vi "数据查询.vi"() -> ()   [LabVIEW 2016, in "数据查询.lvlib"]
uses:
  <vilib>/Utility/miscctls.llb/LVPointTypeDef.ctl
panel:
  in  "标识说明":bool
  in  "数据查询菜单":enum32{"数据查询", "仪器数据", "仪器日志", "报警信息", "校准日志"}(xcontrol)
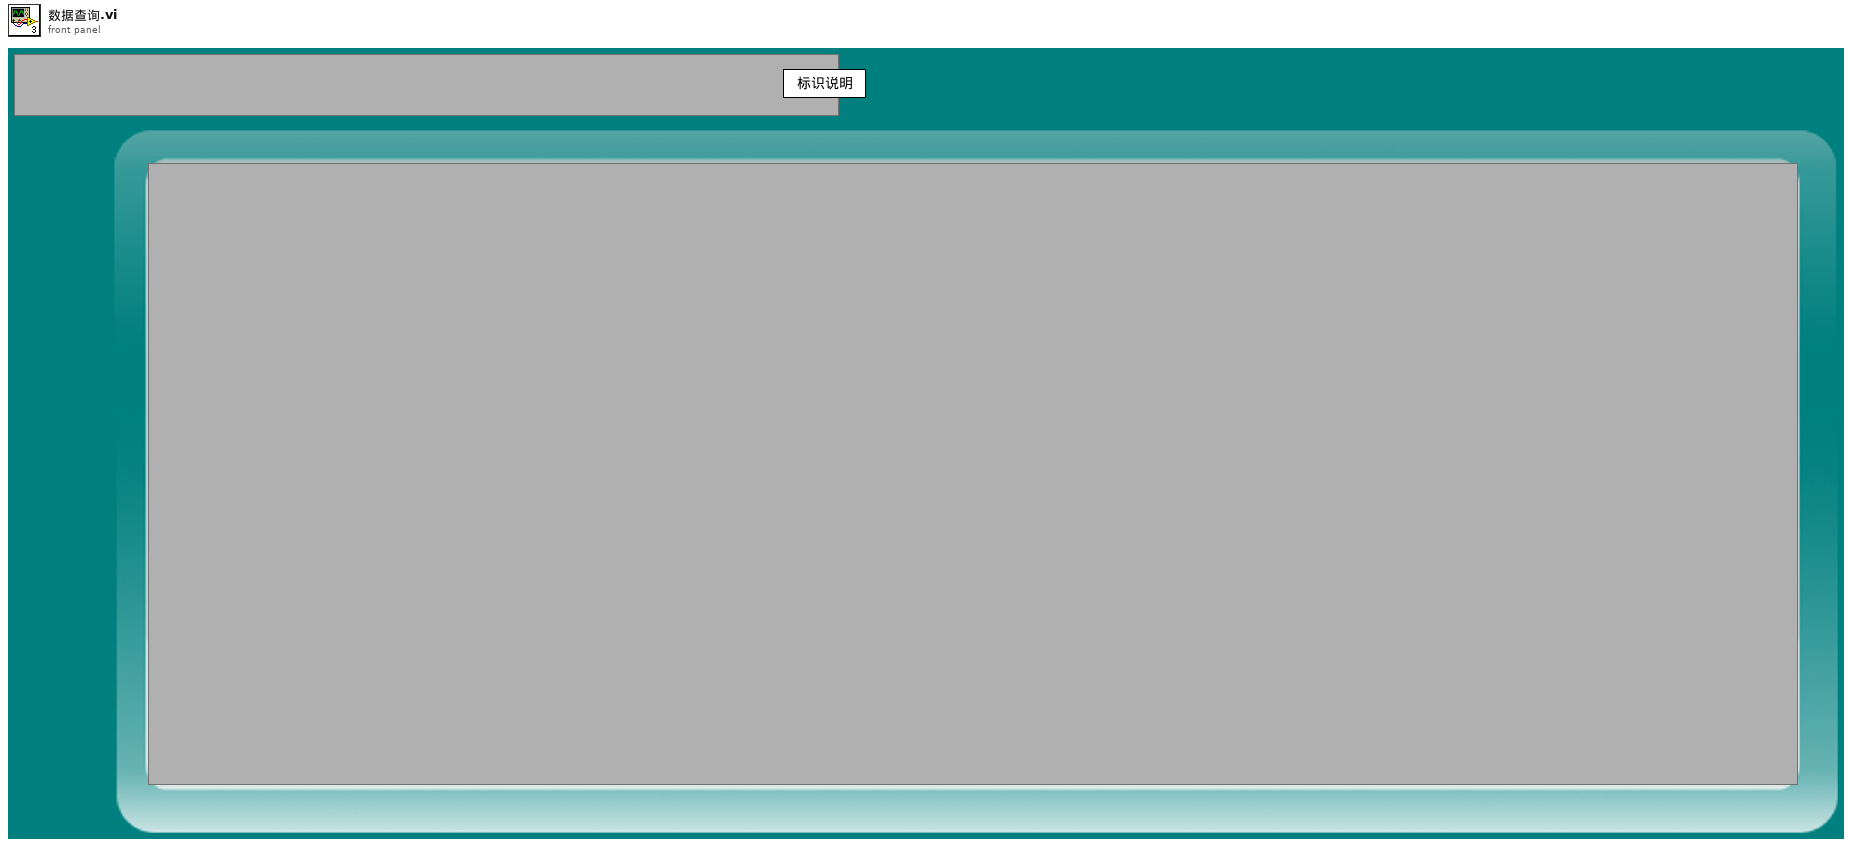
[diagram p1: front panel]
types:
  T1 = typedef "LVPointTypeDef.ctl" = cluster{"Horizontal":i16, "Vertical":i16}
  T2 = enum32{"Bad", "Idle", "Run top level", "Running"}
  T3 = typedef "LVDateTimeRec.ctl" = cluster{"秒数的小数部分":dbl, "秒":i32, "分":i32, "时":i32, "日":i32, "月":i32, "年":i32, "天数（周）":i32, "天数（年）":i32, "DST":i32}
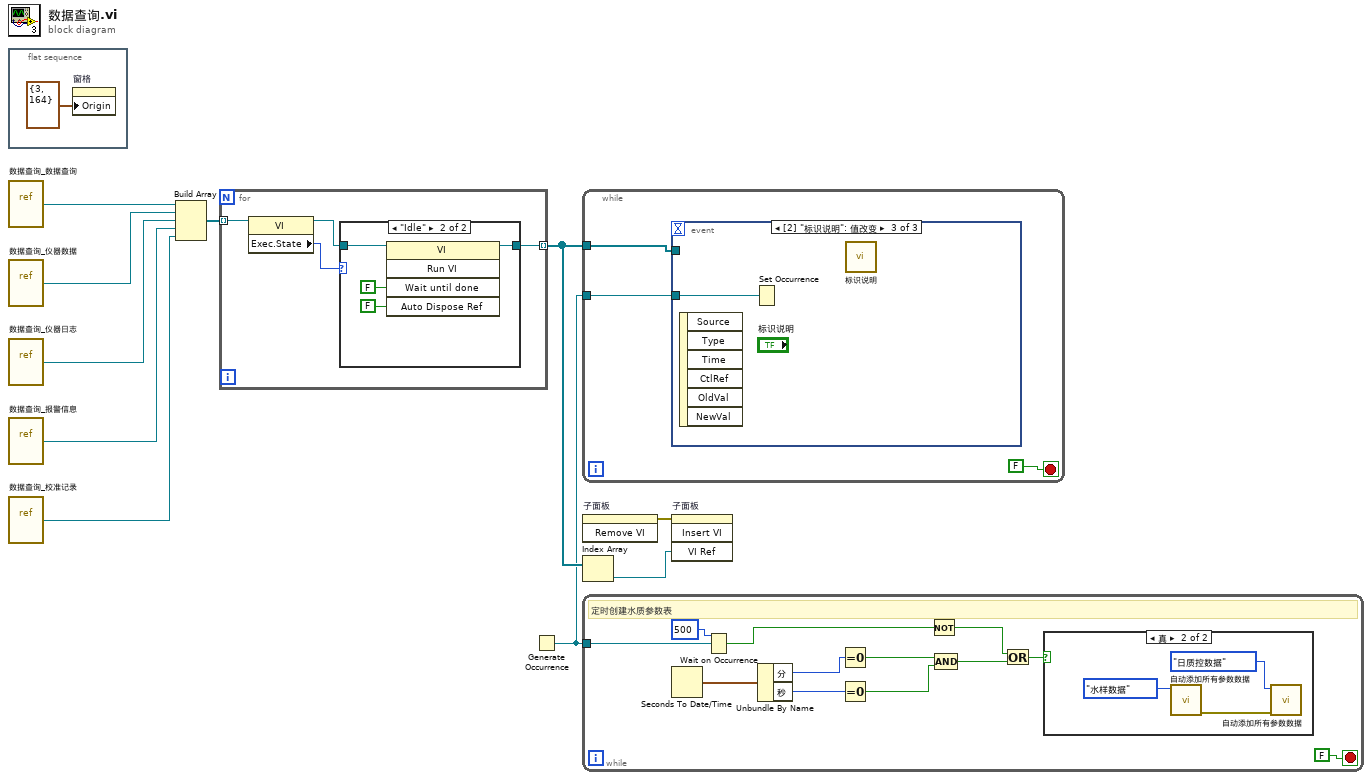
[diagram p0: block diagram]
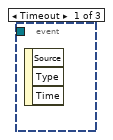
[diagram p4: hidden frame]
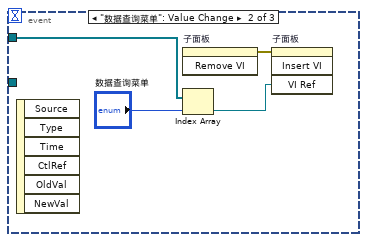
[diagram p5: hidden frame]
diagram:
  n1 = flat-sequence {
    frame #0 {
      n2 = property on="窗格" class="Pane"("Origin"=T1 {"Horizontal"=3, "Vertical"=164} ("原点")) -> ()  [unwired: 2 in, 2 out]
    }
  }
  n3 = vi-ref "数据查询_数据查询.vi"() -> (w7:refnum<vi>)
  n4 = vi-ref "数据查询_仪器数据.vi"() -> (w5:refnum<vi>)
  n5 = vi-ref "数据查询_仪器日志.vi"() -> (w4:refnum<vi>)
  n6 = vi-ref "数据查询_报警信息.vi"() -> (w3:refnum<vi>)
  n7 = vi-ref "数据查询_校准记录.vi"() -> (w2:refnum<vi>)
  n8 = Build Array(w7, w5, w4, w3, w2) -> (w6:refnum<vi>[])
  n9 = for {
    tunnel: w6 -> [w15] mode=indexing
    tunnel: [w12] -> w9 mode=indexing
    n10 = property class="VI"(reference=w15) -> (reference out=w13:refnum<vi>, "Exec.State"=w14:T2)  [unwired: 1 in, 1 out]
    n11 = case shown="\"Idle\"" w14 {
      tunnel: w13 -> [w16 w18]
      tunnel: [w16 w17] -> w12
      frame "Bad", Default {
      }
      frame "Idle" {
        n12 = invoke class="VI" method="Run VI"(reference=w18, "Wait until done"=FALSE ("结束前等待"), "Auto Dispose Ref"=FALSE ("自动销毁引用")) -> (reference out=w17:refnum<vi>)  [unwired: 2 in, 4 out]
      }
    }
  }
  n13 = Generate Occurrence() -> (w1:refnum<k4>)
  n14 = while {
    tunnel: w9 -> [w22]
    tunnel: w1 -> [w21]
    stop <- FALSE stop-if-true
    n15 = event shown="[2] \"标识说明\": 值改变" {
      selector: _ -> [_ _ _]
      dyn-events: _ -> [_ _ _]
      timeout: _ -> [_ _ _]
      tunnel: w22 -> [_ w27 _]
      tunnel: w21 -> [_ _ w28]
      event Timeout {
        n16 = event-data() -> ()  [unwired: 1 in, 3 out]
      }
      event "数据查询菜单": Value Change {
        n17 = event-data() -> ()  [unwired: 1 in, 6 out]
        n18 = invoke on="子面板" class="SubPnl" method="Remove VI"() -> (error out=w24:errorcluster)  [unwired: 3 in, 2 out]
        n19 = Index Array(array=w27, index="数据查询菜单") -> (element=w25:refnum<vi>)
        n20 = invoke on="子面板" class="SubPnl" method="Insert VI"(error in=w24, "VI Ref"=w25) -> ()  [unwired: 2 in, 4 out]
      }
      event "标识说明": Value Change {
        n21 = event-data() -> ()  [unwired: 1 in, 6 out]
        n22 = Set Occurrence(w28) -> ()
        n23 = call "标识说明.vi"() -> ()  [unwired: 12 in]
      }
    }
  }
  n24 = invoke on="子面板" class="SubPnl" method="Remove VI"() -> (error out=w10:errorcluster)  [unwired: 3 in, 2 out]
  n25 = Index Array(array=w9) -> (element=w8:refnum<vi>)  [unwired: 1 in]
  n26 = while {
    tunnel: w1 -> [w33]
    stop <- FALSE stop-if-true
    # "定时创建水质参数表"
    n27 = Seconds To Date/Time() -> (date time rec=w40:T3)  [unwired: 2 in]
    n28 = Wait on Occurrence(2:w33, 3:500 ("毫秒超时(-1)")) -> (0:w30:bool)  [unwired: 1 in]
    n29 = Unbundle By Name(w40) -> ("分"=w39:i32, "秒"=w38:i32)
    n30 = Equal To 0?(x=w39) -> (x = 0?=w37:bool)
    n31 = Equal To 0?(x=w38) -> (x = 0?=w36:bool)
    n32 = Not(x=w30) -> (.not. x?=w29:bool)
    n33 = Compound Arithmetic op=AND ("复合运算")(w37, w36) -> (w35:bool)
    n34 = Or(x=w29, y=w35) -> (x .or. y?=w31:bool)
    n35 = case shown="真" w31 {
      frame False {
      }
      frame True {
        n36 = call "自动添加所有参数数据.vi"("数据类别"=enum16{"水样数据", "日质控数据"}."水样数据") -> ("错误输出"=w43:errorcluster)  [unwired: 10 in]
        n37 = call "自动添加所有参数数据.vi"("error in (no error)"=w43, "数据类别"=enum16{"水样数据", "日质控数据"}."日质控数据") -> ()  [unwired: 9 in, 1 out]
      }
    }
  }
  n38 = invoke on="子面板" class="SubPnl" method="Insert VI"(error in=w10, "VI Ref"=w8) -> ()  [unwired: 2 in, 4 out]
